vi "Get Enable State.vi"(8 "error in (no error)":errorcluster, 11 "logger name":string) -> (0 "error out":errorcluster, 3 "enabled?":bool)   [LabVIEW 2018, in "GLog.lvlib" / "Registry.lvlib"]
uses:
  Registry.lvlib
  Registry Actions.ctl
  reuse_library/Utilities/Utilities.lvlib
panel:
  # "Connector Pane"
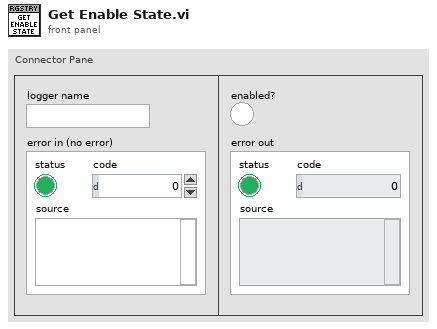
[diagram p1: front panel]
types:
  T1 = cluster{"Enabled?":bool, "error out":errorcluster}
  T2 = typedef "GLog.lvlib/Registry.lvlib/Registry Actions.ctl" = enum16{"Register", "Log", "Enable", "Enable All", "Disable", "Disable All", "Get Enable State", "Get Minimum Log Level", "Set Minimum Log Level", "Set All Minimum Log Level", "Get Logger Info", "Get All Logger Info", "List", "Unregister", "Unregister All", "Shutdown"}
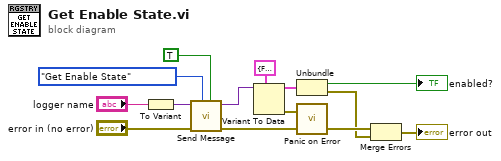
[diagram p0: block diagram]
diagram:
  n1 = To Variant(anything="logger name") -> (Variant=w10:variant)
  n2 = call "Send Message.vi"("return data? (F)"=TRUE, "action"=Registry_Actions."Get Enable State", "error in (no error)"="error in (no error)", "send data"=w10) -> ("error out"=w13:errorcluster, "return data"=w8:variant)  [unwired: 6 in]
  n3 = Variant To Data(type=T1 {"Enabled?"=FALSE, "error out"={"status"=FALSE, "code"=0, "source"=""}}, Variant=w8) -> (data=w3:T1, error out=w7:errorcluster)  [unwired: 1 in]
  n4 = Unbundle(w3) -> ("Enabled?"=→"enabled?":bool, "error out"=w2:errorcluster)
  n5 = call "Panic on Error.vi"("error in (no error)"=w7) -> ()  [unwired: 3 in]
  n6 = Merge Errors(w13, w2) -> (→"error out":errorcluster)
